vi "Example_Cluster_Payload.vi"() -> ()   [LabVIEW 2020, in "PixPack.lvlib"]
uses:
  PixPack.lvlib
  private/Encode.Format.ctl
  private/User.Encode.Format.ctl
  ce672bd1-fffe-424f-a641-cc0b68ed6e9e.vi
  <vilib>/Utility/error.llb/Clear Errors.vi
  private/PP.ReadFile.To.ByteArray.vi
  private/Get.Flatten.TypeAndData.vi
  <vilib>/Utility/error.llb/Error Cluster From Error Code.vi
  <vilib>/Utility/libraryn.llb/Generate Temporary File Path.vi
  private/PP.Create.File.By.ByteArray.vi
  <vilib>/picture/png.llb/Read PNG File.vi
  <vilib>/wsapi/VIs/PNG Data to LV Image.vi
panel:
  out "Type of Encode":T1=enum."PIX_EXT_FILE"
  out "2D Picture":picture
  out "error out":errorcluster
  out "XML Out (if XML Flattened)":string
  out "Value":T2(array[cluster])
  in  "error in":errorcluster
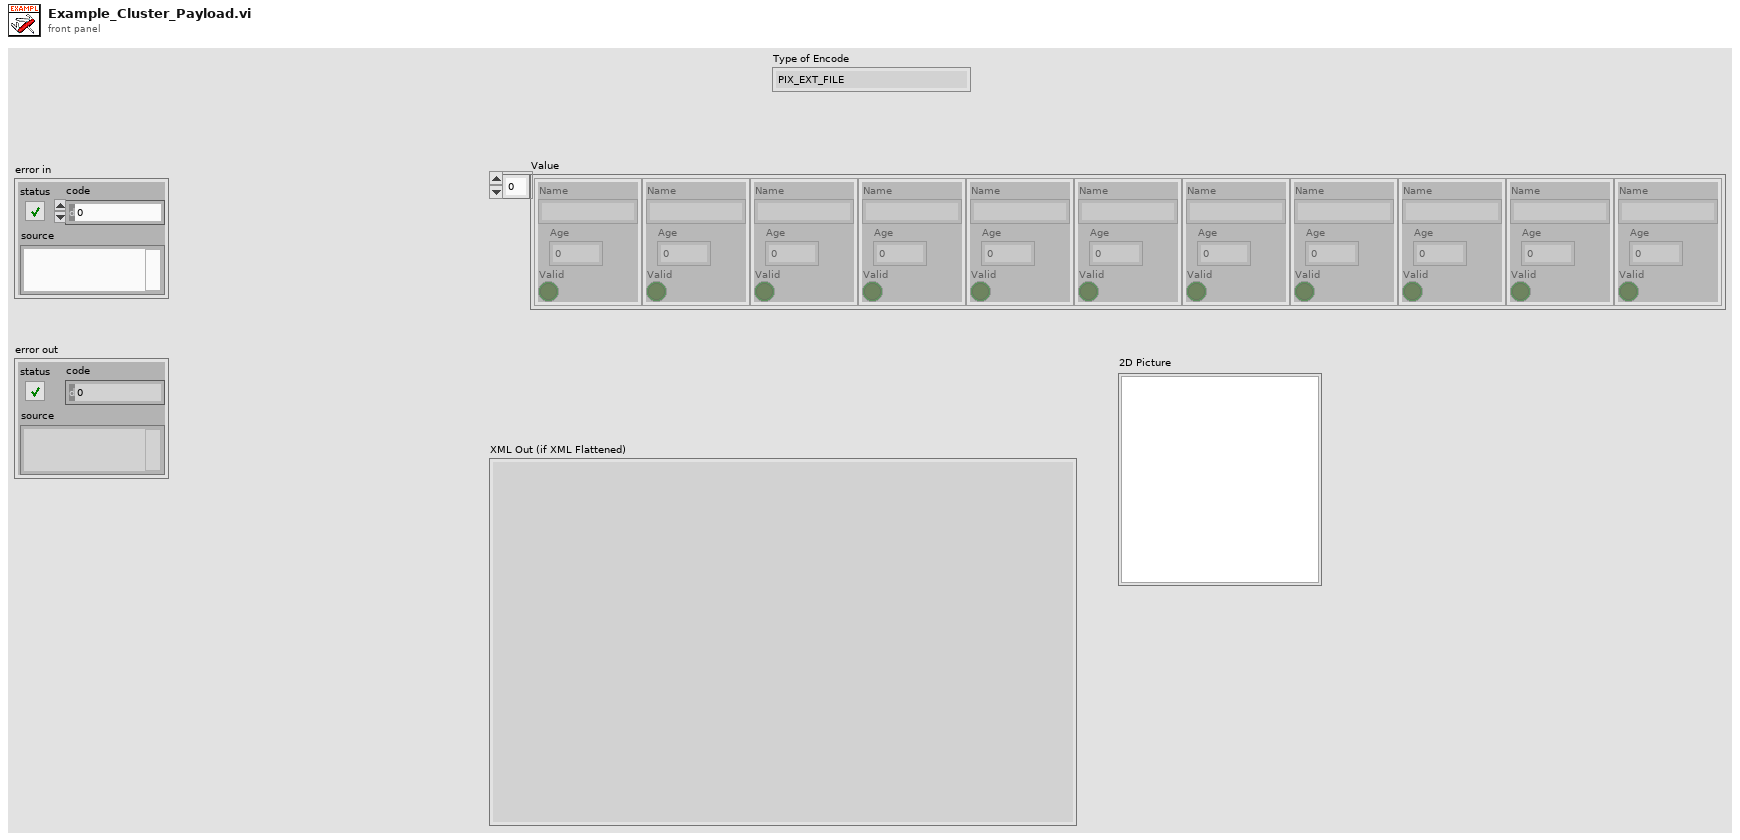
[diagram p1: front panel]
types:
  T1 = typedef "PixPack.lvlib/Encode.Format.ctl" = enum16{"PIX_NOR_FLAT", "PIX_XFLAT", "PIX_EXT_FILE", "PIX_NOT_ENCODED"}
  T2 = cluster{"Name":string, "Age":i32, "Valid":bool}[]
  T3 = typedef "PixPack.lvlib/User.Encode.Format.ctl" = enum16{"XML Encode", "Normal Flatten", "External File"}
  T4 = typedef "imagedata.ctl" = cluster{"image type":i32, "image depth":i32, "image":u8[], "mask":u8[], "colors":u32[], "Rectangle":cluster{"left":i16, "top":i16, "right":i16, "bottom":i16}}
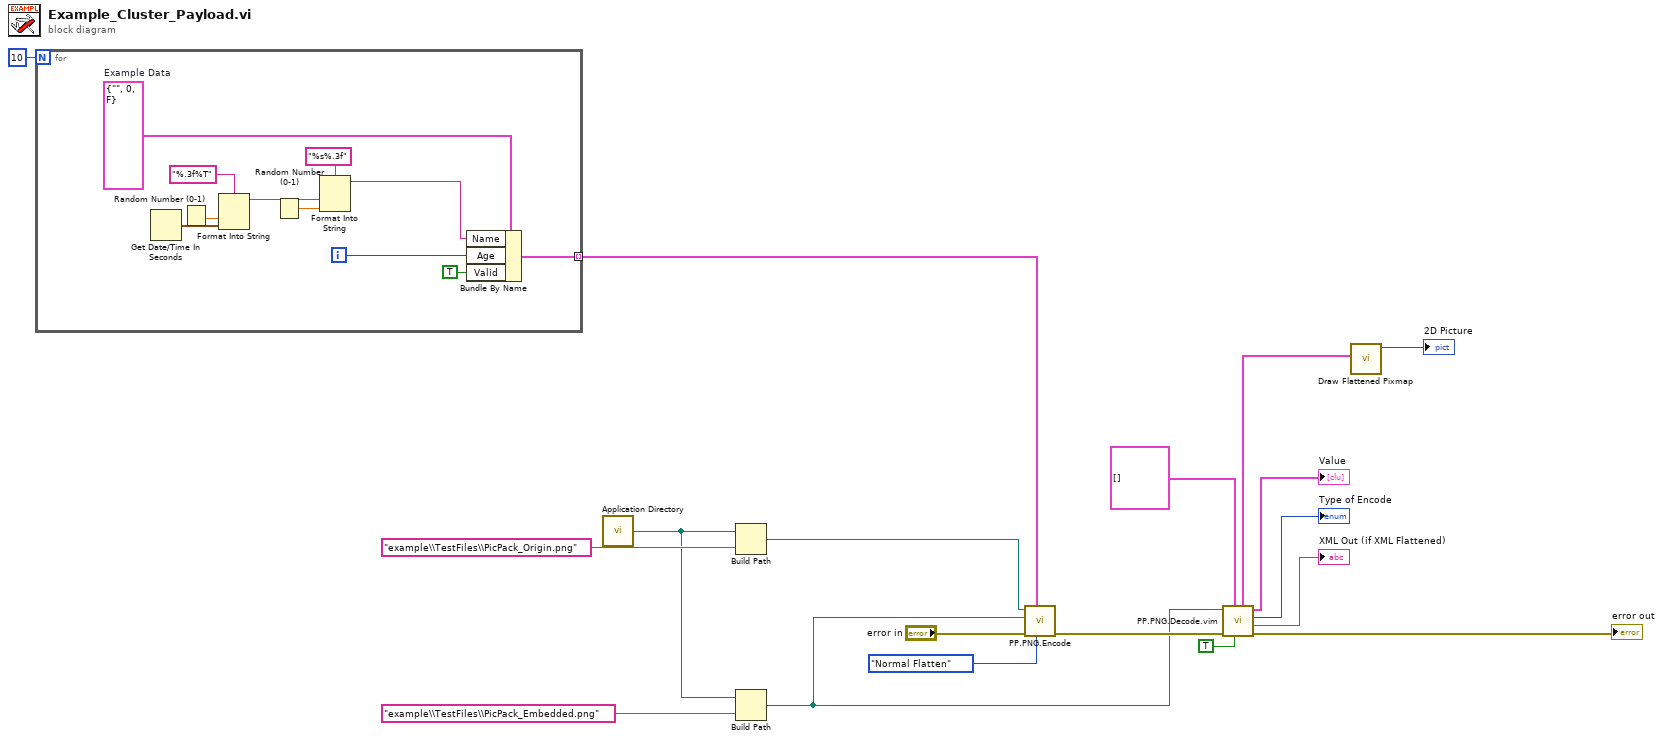
[diagram p0: block diagram]
diagram:
  n1 = for {
    N: 10 -> [_]
    tunnel: [w19] -> w1 mode=indexing
    i -> [w21]
    w23 = cluster{"Name":string, "Age":i32, "Valid":bool} {"Name"="", "Age"=0, "Valid"=FALSE}  # Example Data
    n2 = Get Date/Time In Seconds() -> (seconds since 1Jan1904=w27:timestamp)
    n3 = Random Number (0-1)() -> (number: 0 to 1=w28:dbl)
    n4 = Format Into String(format string="%.3f%T", w28, w27) -> (resulting string=w29:string)  [unwired: 2 in, 1 out]
    n5 = Random Number (0-1)() -> (number: 0 to 1=w24:dbl)
    n6 = Format Into String(format string="%s%.3f", w29, w24) -> (resulting string=w22:string)  [unwired: 2 in, 1 out]
    n7 = Bundle By Name(cluster=w23, "Name"=w22, "Age"=w21, "Valid"=TRUE) -> (w19:cluster{"Name":string, "Age":i32, "Valid":bool})
  }
  n8 = call <vilib>:"Application Directory.vi"() -> ("Application Directory"=w9:path)
  n9 = Build Path(base path=w9, name or relative path="example\\TestFiles\\PicPack_Origin.png") -> (appended path=w5:path)
  n10 = Build Path(base path=w9, name or relative path="example\\TestFiles\\PicPack_Embedded.png") -> (appended path=w4:path)
  n11 = call "PP.PNG.Encode.vi"("Encode Format"=User.Encode.Format."Normal Flatten", "Data"=w1, "error in"="error in", "Destination PNG (default: empty)"=w4, "PNG In"=w5) -> ("error out"=w16:errorcluster)  [unwired: 6 in]
  n12 = call "PP.PNG.Decode.vim"("Get Image Data (F)"=TRUE, "Data Type (Default)"=T2 [] ("appended array"), "error in"=w16, "PNG In"=w4) -> ("error out"=→"error out":errorcluster, "XML Out (if XML Flattened)"=→"XML Out (if XML Flattened)":string, "Type of Encode"=→"Type of Encode":T1, "Value"=→"Value":T2, "Image Data"=w12:T4)  [unwired: 3 in]
  n13 = call <vilib>:"Draw Flattened Pixmap.vi"("image data"=w12) -> ("new picture"=→"2D Picture":picture)  [unwired: 8 in]
